vi "Parse XML Elements.vi"(0 "DOM":refnum<k20>) -> ()   [LabVIEW 2013]
uses:
  <resource>/objmgr/DOMUserDefRef.rc
  <vilib>/xml/NI_XML.lvlib
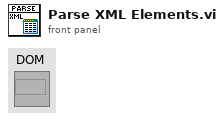
[diagram p1: front panel]
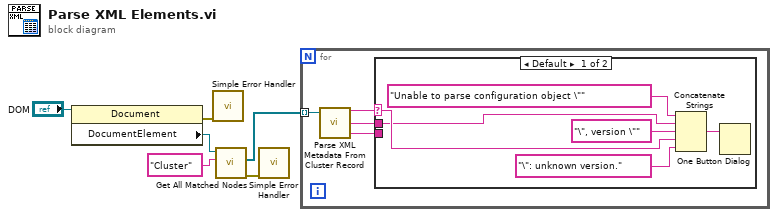
[diagram p0: block diagram]
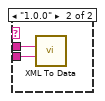
[diagram p2: hidden frame]
diagram:
  n1 = property class="Document"(reference="DOM") -> (error out=w5:errorcluster, "DocumentElement"=w3:refnum<k20>)  [unwired: 1 in, 1 out]
  n2 = call <vilib>:"Simple Error Handler.vi"("error in (no error)"=w5) -> ()  [unwired: 4 in, 5 out]
  n3 = call <vilib>:"Get All Matched Nodes.vi"("XPath expression"="Cluster" ("Tag Name"), "node in"=w3) -> ("error out"=w2:errorcluster, "node result array"=w1:refnum<k20>[])  [unwired: 7 in, 1 out]
  n4 = call <vilib>:"Simple Error Handler.vi"("error in (no error)"=w2) -> ()  [unwired: 4 in, 5 out]
  n5 = for {
    tunnel: w1 -> [w10] mode=indexing
    n6 = call "Parse XML Metadata From Cluster Record.vi"("Node Reference"=w10) -> ("XML Data"=w7:string, "Name"=w9:string, "Version"=w8:string)  [unwired: 2 in]
    n7 = case shown="Default" w8 {
      selector: w8 -> [w14 _]
      tunnel: w9 -> [w11 w18]
      tunnel: w7 -> [_ w17]
      frame Default {
        n8 = Concatenate Strings("Unable to parse configuration object \"" ("string"), w11, "\", version \"" ("string"), w14, "\": unknown version." ("string")) -> (w12:string)
        n9 = One Button Dialog(message=w12) -> ()  [unwired: 1 in, 1 out]
      }
      frame "1.0.0" {
        n10 = call "XML To Data.vi"("XML Data"=w17, "Name"=w18) -> ()  [unwired: 1 in]
      }
    }
  }
